vi "measure_volt_dc.vi"(8 "error in (no error)":errorcluster, 10 "UI out 3":T8, 11 "paramUnicorn in":T1) -> (0 "error out":errorcluster, 1 "measured":dbl[](array[numeric]), 2 "UI out 2":T8, 3 "paramUnicorn 2":T1, 5 "boc_data":sgl[](array[numeric]))   [LabVIEW 2017]
uses:
  ui.ctl
  classes/dc_power_supply/DC_power_supply.lvclass
  classes/report/Report.lvclass
  ui_buttons.ctl
  types/boc_type.ctl
  Unicorn Labview Library/Control/unicorn_Param.ctl
  Unicorn Labview Library/Control/unicorn_conn.ctl
  Unicorn Labview Library/Control/unicorn_JSON.ctl
  Unicorn Labview Library/Control/unicorn_ParamInt.ctl
  Unicorn Labview Library/Control/unicorn_Telemetry.ctl
  Unicorn Labview Library/Control/unicorn_Table.ctl
  Unicorn Labview Library/Control/unicorn_ParamFloat.ctl
  <instrlib>/PICOTEST M352XA/Public/Controls/Function.ctl
  Unicorn Labview Library/Unicorn Library.lvlib
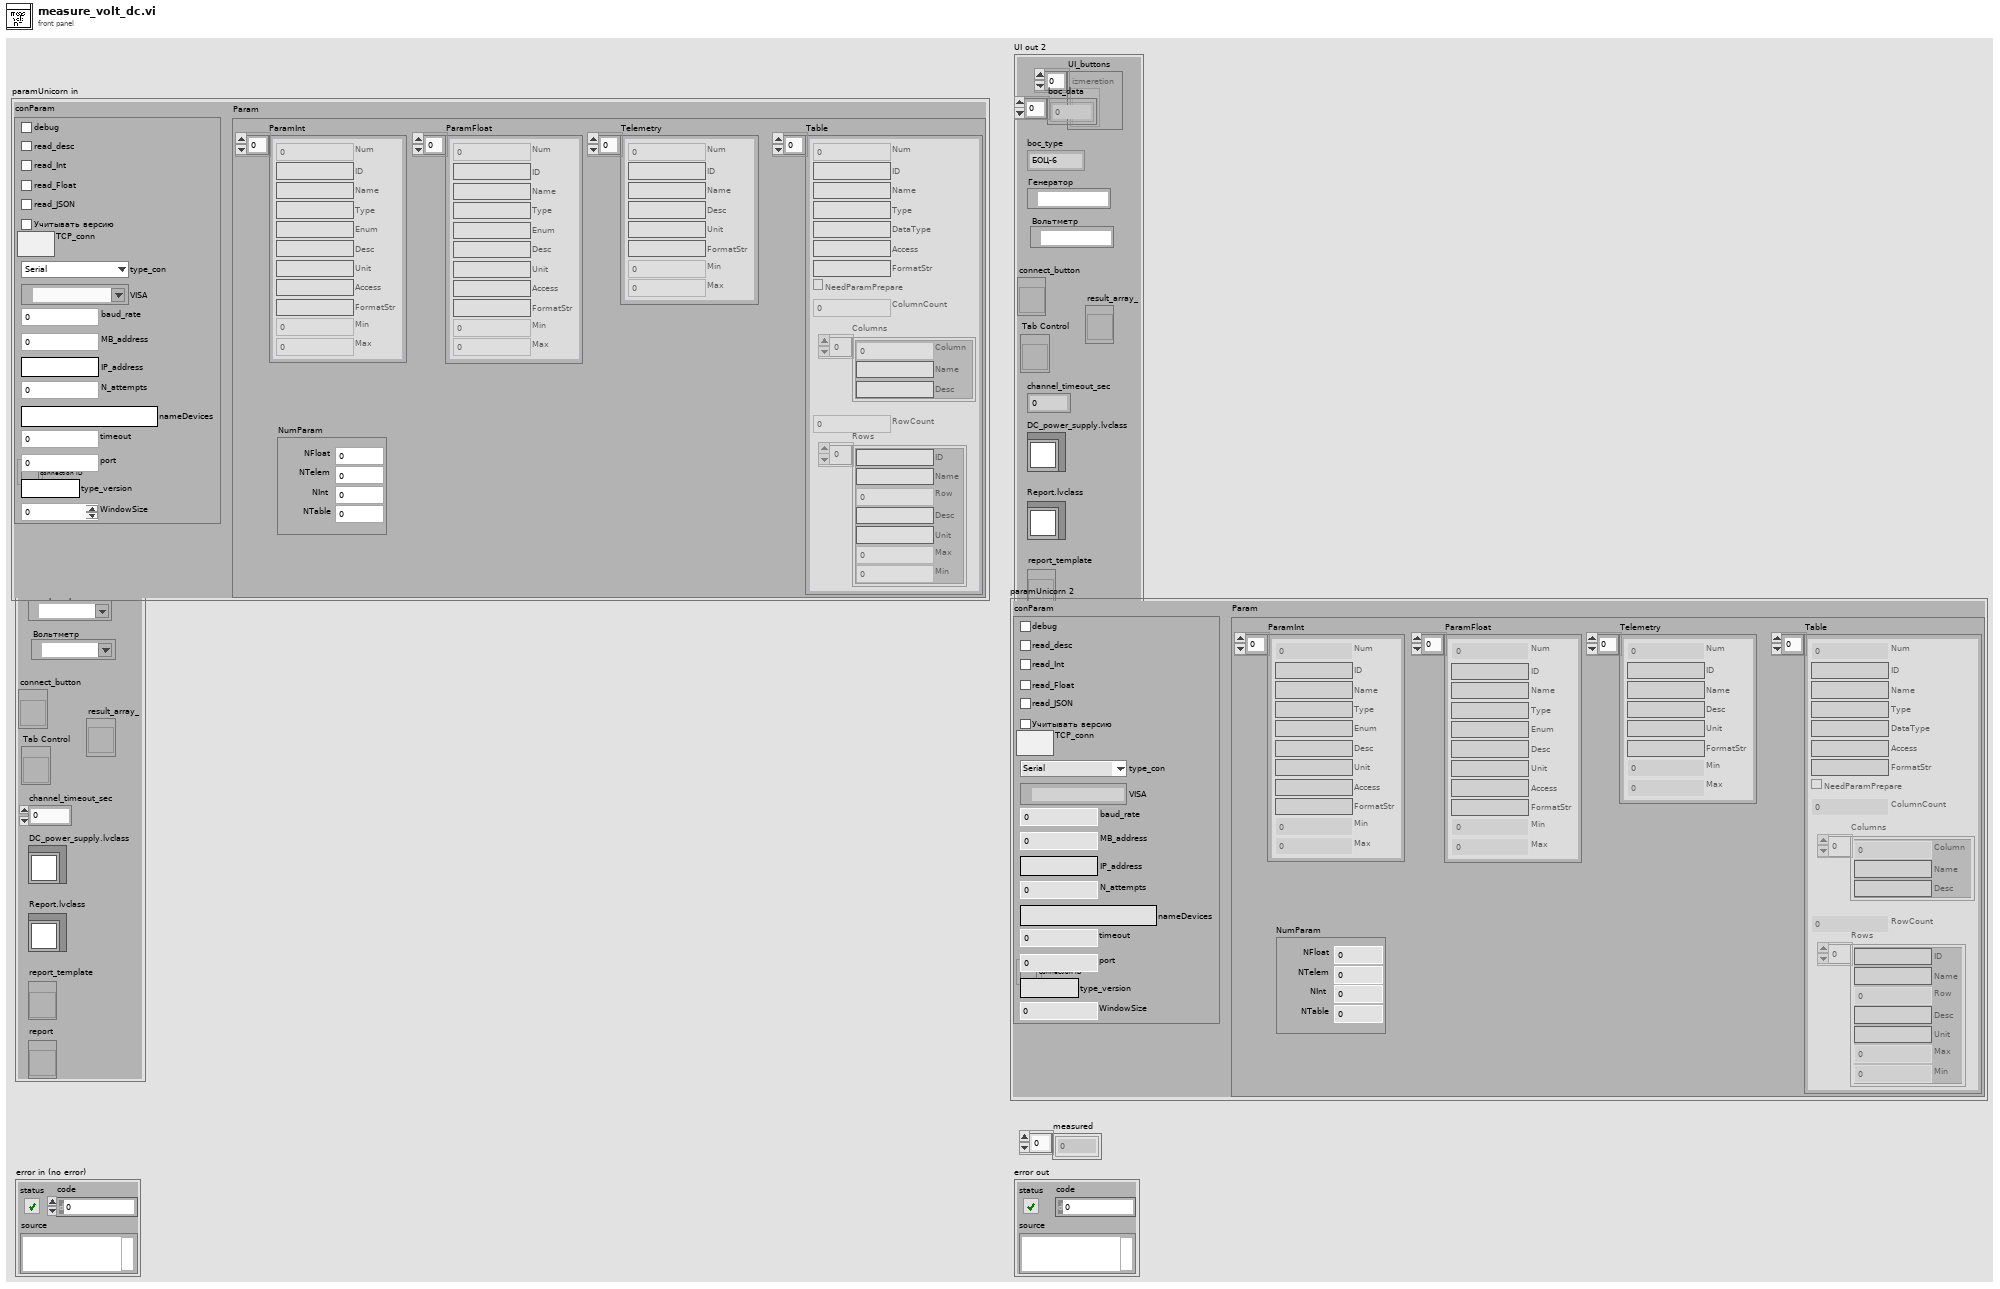
[diagram p1: front panel]
types:
  T1 = typedef "Unicorn Library.lvlib/unicorn_Param.ctl" = cluster{"conParam":T2, "Param":T3}
  T2 = typedef "Unicorn Library.lvlib/unicorn_conn.ctl" = cluster{"ReadIntParam":bool, "ReadDescrParam":bool, "ReadFloatParam":bool, "debug":bool, "ReadJSON":bool, "IP_address":string, "N_attempts":i32, "type_con":enum16{"Serial", "TCP"}, "MB_address":i32, "VISA":refnum<visa-resource-name>, "connection ID":refnum<k5>, "nameDevices":string, "timeout":i32, "port":u16, "type_version":string, "baud_rate":u32, "VersionControl":bool, "TCP_conn":bool, "WindowSize":i32}
  T3 = typedef "Unicorn Library.lvlib/unicorn_JSON.ctl" = cluster{"NumParam":cluster{"NTelem":i32, "NInt":i32, "NFloat":i32, "NTable":i32}, "ParamInt":T4, "Telemetry":T5, "Table":T6, "ParamFloat":T7}
  T4 = typedef "Unicorn Library.lvlib/unicorn_ParamInt.ctl" = cluster{"ID":string, "Num":i32, "Name":string, "Type":string, "Enum":string, "Desc":string, "Unit":string, "Access":string, "FormatStr":string, "Min":i32, "Max":i32}[]
  T5 = typedef "Unicorn Library.lvlib/unicorn_Telemetry.ctl" = cluster{"ID":string, "Num":i32, "Name":string, "Desc":string, "Unit":string, "FormatStr":string, "Min":i32, "Max":i32}[]
  T6 = typedef "Unicorn Library.lvlib/unicorn_Table.ctl" = cluster{"Num":i32, "Access":string, "ColumnCount":i32, "NeedParamPrepare":bool, "Columns":cluster{"Column":i32, "Desc":string, "Name":string}[], "DataType":string, "FormatStr":string, "ID":string, "Name":string, "RowCount":i32, "Rows":cluster{"Desc":string, "ID":string, "Max":i32, "Min":i32, "Name":string, "Row":i32, "Unit":string}[], "Type":string}[]
  T7 = typedef "Unicorn Library.lvlib/unicorn_ParamFloat.ctl" = cluster{"ID":string, "Num":i32, "Name":string, "Type":string, "Enum":string, "Desc":string, "Unit":string, "Access":string, "FormatStr":string, "Min":i32, "Max":i32}[]
  T8 = typedef "ui.ctl" = cluster{"UI_buttons":T9, "Tab Control":refnum<vi>, "connect_button":refnum<vi>, "generator":refnum<visa-resource-name>, "voltmetr":refnum<visa-resource-name>, "channel_timeout_sec":dbl, "boc_type":T10, "result_array_":refnum<vi>, "DC_power_supply.lvclass":refnum<class "DC_power_supply.lvclass">, "Report.lvclass":refnum<class "Report.lvclass">, "report_template":refnum<vi>, "report":refnum<vi>}
  T9 = typedef "ui_buttons.ctl" = refnum<vi>[]
  T10 = typedef "boc_type.ctl" = enum16{"БОЦ-6", "БОЦ-12"}
  T11 = typedef "Function.ctl" = enum16{"VOLTage:DC", "VOLTage:DC:RATio", "VOLTage:AC", "CURRent:DC", "CURRent:AC", "RESistance", "FRESistance", "FREQuency", "PERiod", "FREQuency:CURRent", "PERiod:CURRent", "CAPacitance", "CONTinuity", "DIODe", "TCOuple", "TEMPerature"}
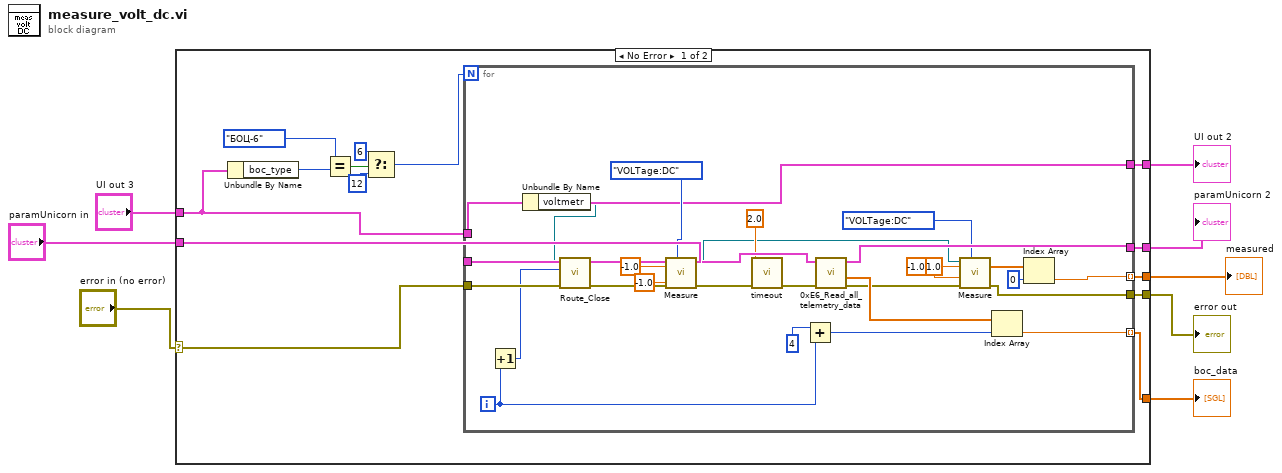
[diagram p0: block diagram]
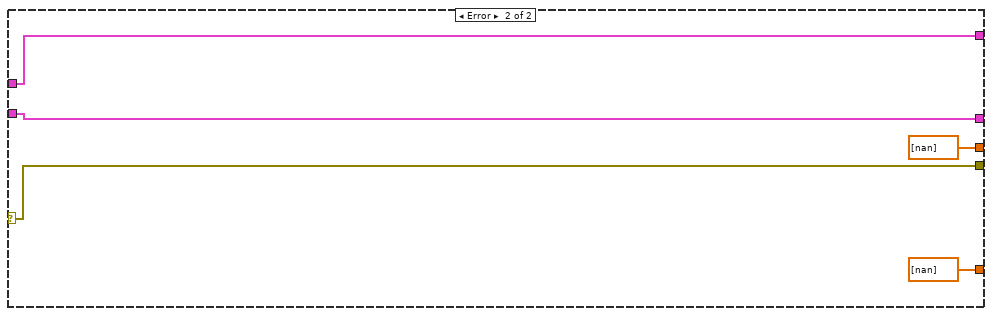
[diagram p2: hidden frame]
diagram:
  n1 = case shown="No Error" "error in (no error)" {
    selector: "error in (no error)" -> [w9 w55]
    tunnel: [w22 w53] -> w8
    tunnel: [w21 w55] -> w7
    tunnel: [w20 sgl[] [nan]] -> w6
    tunnel: [w19 dbl[] [nan]] -> w5
    tunnel: [w18 w54] -> w4
    tunnel: "paramUnicorn in" -> [w17 w54]
    tunnel: "UI out 3" -> [w16 w53]
    frame No Error {
      n2 = Unbundle By Name(w16) -> ("boc_type"=w15:T10)
      n3 = Equal?(x=boc_type."БОЦ-6", y=w15) -> (x = y?=w13:bool)
      n4 = Select(t=u8 6, s=w13, f=u8 12) -> (s? t:f=w10:u8)
      n5 = for {
        N: w10 -> [_]
        tunnel: w16 -> [w26]
        tunnel: w9 -> [w48]
        tunnel: [w44] -> w20 mode=indexing
        tunnel: w17 -> [w50]
        tunnel: [w49] -> w18
        tunnel: [w23] -> w19 mode=indexing
        tunnel: [w35] -> w21
        tunnel: [w26] -> w22
        i -> [w43]
        n6 = Increment(x=w43) -> (x+1=w29:i32)
        n7 = Unbundle By Name(w26) -> ("voltmetr"=w25:refnum<visa-resource-name>)
        n8 = call <instrlib>:"Route_Close.vi"("error in (no error)"=w48, "channel"=w29, "VISA resource name"=w25) -> ("error out"=w40:errorcluster, "VISA resource name out"=w39:refnum<visa-resource-name>)  [unwired: 6 in, 1 out]
        n9 = call <instrlib>:"Measure.vi"("Function"=Function."VOLTage:DC", "error in (no error)"=w40, "Resolution"=-1.0, "Range"=-1.0, "VISA resource name"=w39) -> ("error out"=w32:errorcluster, "VISA resource name out"=w24:refnum<visa-resource-name>)  [unwired: 4 in, 1 out]
        n10 = call "timeout.vi"("error in (no error)"=w32, "seconds to wait"=2.0) -> ("error IO"=w42:errorcluster)  [unwired: 9 in]
        n11 = Add(x=4, y=w43) -> (x+y=w45:i32)
        n12 = call "0xE6_Read_all_telemetry_data.vi"("error in"=w42, "paramUnicorn"=w50) -> ("error out"=w38:errorcluster, "Telemetry"=w46:sgl[], "paramUnicorn 2"=w49:T1)  [unwired: 5 in, 1 out]
        n13 = call <instrlib>:"Measure.vi"("Function"=Function."VOLTage:DC", "error in (no error)"=w38, "Resolution"=-1.0, "Range"=-1.0, "VISA resource name"=w24) -> ("error out"=w35:errorcluster, "Measurements"=w34:dbl[])  [unwired: 4 in, 1 out]
        n14 = Index Array(array=w46, index=w45) -> (element=w44:sgl)
        n15 = Index Array(array=w34, index=0) -> (element=w23:dbl)
      }
    }
    frame Error {
    }
  }
  "UI out 2" <- w8
  "error out" <- w7
  "boc_data" <- w6
  "measured" <- w5
  "paramUnicorn 2" <- w4
